vi "New One-Shot Subscription.vi"(10 "Ignore Past Updates? (F)":bool, 11 "OneShotSubscription In":refnum<class "OneShotSubscription.lvclass">) -> (3 "OneShotSubscription Out":refnum<class "OneShotSubscription.lvclass">)   [LabVIEW 2018, in "MVA Framework.lvlib" / "SubscriptionPolicy.lvlib" / "OneShotSubscription.lvclass"]
doc: "新建一次性订阅"
uses:
  OneShotSubscription.lvclass
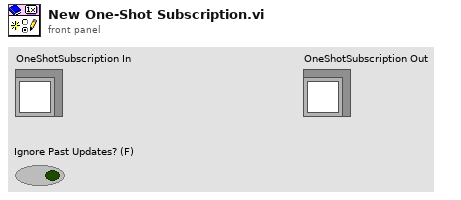
[diagram p1: front panel]
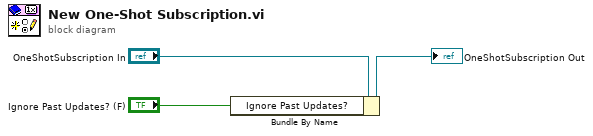
[diagram p0: block diagram]
diagram:
  n1 = Bundle By Name(cluster="OneShotSubscription In", "Ignore Past Updates?"="Ignore Past Updates? (F)") -> (→"OneShotSubscription Out":refnum<class "OneShotSubscription.lvclass">)
